vi "大富翁.vi"() -> ()   [LabVIEW 2014] (continued)
                      frame 1, Default {
                        n4206 = local read "玩家一財產"() -> (w3544:dbl)
                      }
                      frame 2 {
                        n4207 = local read "玩家二財產"() -> (w3545:dbl)
                      }
                      frame 3 {
                        n4208 = local read "玩家三財產"() -> (w3546:dbl)
                      }
                      frame 4 {
                        n4209 = local read "玩家四財產"() -> (w3547:dbl)
                      }
                    }
                    n4210 = call "各種價格.vi"("Numeric"=w3516) -> ("買空地"=w3514:dbl)  [unwired: 4 in, 5 out]
                    n4211 = Greater Or Equal?(x=w3515, y=w3514) -> (x >= y?=w3513:bool)
                    n4212 = case shown="True" w3513 {
                      tunnel: w3516 -> [_ w3518]
                      frame False {
                        # "錢不夠"
                        n4213 = call "錢不夠.vi"() -> ()  [unwired: 4 in]
                      }
                      frame True {
                        # "錢夠"
                        n4214 = local read "換誰?"() -> (w3519:dbl)
                        n4215 = case shown="3" w3519 {
                          selector: w3519 -> [w3523 w3529 w3535 w3541]
                          tunnel: w3518 -> [w3522 w3528 w3534 w3540]
                          frame 1, Default {
                            # "誰買了地"
                            n4216 = call "各種價格.vi"("Numeric"=w3522) -> ("買空地"=w3521:dbl)  [unwired: 4 in, 5 out]
                            n4217 = local read "玩家一財產"() -> (w3525:dbl)
                            n4218 = Subtract(x=w3525, y=w3521) -> (x-y=w3524:dbl)
                            n4219 = local write "玩家一財產"(w3524) -> ()
                            n4220 = call "數字轉顏色.vi"("數字"=w3523) -> ("顏色數字"=w3520:dbl)  [unwired: 2 in]
                            n4221 = local write "34新竹縣"(w3520) -> ()
                            n4222 = local write "新竹縣所有"(w3520) -> ()
                          }
                          frame 2 {
                            # "誰買了地"
                            n4223 = call "各種價格.vi"("Numeric"=w3528) -> ("買空地"=w3527:dbl)  [unwired: 4 in, 5 out]
                            n4224 = local read "玩家二財產"() -> (w3531:dbl)
                            n4225 = Subtract(x=w3531, y=w3527) -> (x-y=w3530:dbl)
                            n4226 = local write "玩家二財產"(w3530) -> ()
                            n4227 = call "數字轉顏色.vi"("數字"=w3529) -> ("顏色數字"=w3526:dbl)  [unwired: 2 in]
                            n4228 = local write "34新竹縣"(w3526) -> ()
                            n4229 = local write "新竹縣所有"(w3526) -> ()
                          }
                          frame 3 {
                            # "誰買了地"
                            n4230 = local read "玩家三財產"() -> (w3536:dbl)
                            n4231 = call "各種價格.vi"("Numeric"=w3534) -> ("買空地"=w3533:dbl)  [unwired: 4 in, 5 out]
                            n4232 = Subtract(x=w3536, y=w3533) -> (x-y=w3537:dbl)
                            n4233 = call "數字轉顏色.vi"("數字"=w3535) -> ("顏色數字"=w3532:dbl)  [unwired: 2 in]
                            n4234 = local write "玩家三財產"(w3537) -> ()
                            n4235 = local write "34新竹縣"(w3532) -> ()
                            n4236 = local write "新竹縣所有"(w3532) -> ()
                          }
                          frame 4 {
                            # "誰買了地"
                            n4237 = call "各種價格.vi"("Numeric"=w3540) -> ("買空地"=w3539:dbl)  [unwired: 4 in, 5 out]
                            n4238 = local read "玩家四財產"() -> (w3543:dbl)
                            n4239 = Subtract(x=w3543, y=w3539) -> (x-y=w3542:dbl)
                            n4240 = local write "玩家四財產"(w3542) -> ()
                            n4241 = call "數字轉顏色.vi"("數字"=w3541) -> ("顏色數字"=w3538:dbl)  [unwired: 2 in]
                            n4242 = local write "34新竹縣"(w3538) -> ()
                            n4243 = local write "新竹縣所有"(w3538) -> ()
                          }
                        }
                      }
                    }
                  }
                }
              }
            }
          }
          frame 36 {
            n4244 = local read "新竹市所有"() -> (w3548:u32)
            n4245 = Equal?(x=w3548, y=u32 16777215) -> (x = y?=w3551:bool)
            n4246 = case shown="False" w3551 {
              tunnel: w3550 -> [w3574 w3612]
              tunnel: [w3564 FALSE] -> w3549
              frame False {
                # "有主地"
                n4247 = local read "換誰?"() -> (w3567:dbl)
                n4248 = local read "新竹市所有"() -> (w3555:u32)
                n4249 = call "數字轉顏色.vi"("數字"=w3567) -> ("顏色數字"=w3578:dbl)  [unwired: 2 in]
                n4250 = case shown="4" w3567 {
                  tunnel: [w3607 w3608 w3609 w3610] -> w3573
                  frame 1, Default {
                    n4251 = local read "玩家一財產"() -> (w3607:dbl)
                  }
                  frame 2 {
                    n4252 = local read "玩家二財產"() -> (w3608:dbl)
                  }
                  frame 3 {
                    n4253 = local read "玩家三財產"() -> (w3609:dbl)
                  }
                  frame 4 {
                    n4254 = local read "玩家四財產"() -> (w3610:dbl)
                  }
                }
                n4255 = Equal?(x=w3555, y=w3578) -> (x = y?=w3577:bool)
                n4256 = local read "36旅4"() -> (w3556:bool)
                n4257 = local read "36旅3"() -> (w3557:bool)
                n4258 = local read "36旅2"() -> (w3558:bool)
                n4259 = local read "36旅1"() -> (w3559:bool)
                n4260 = local read "36房4"() -> (w3560:bool)
                n4261 = local read "36房3"() -> (w3561:bool)
                n4262 = local read "36房2"() -> (w3562:bool)
                n4263 = local read "36房1"() -> (w3563:bool)
                n4264 = local read "新竹市所有"() -> (w3554:u32)
                n4265 = call "房子數量.vi"("房子 1"=w3563, "房子 2"=w3562, "房子 3"=w3561, "房子 4"=w3560, "旅館 1"=w3559, "旅館 2"=w3558, "旅館 3"=w3557, "旅館 4"=w3556) -> ("房子數"=w3576:dbl, "旅館數"=w3575:dbl)  [unwired: 18 in]
                n4266 = call "顏色轉數字.vi"("顏色數字"=w3554) -> ("數字"=w3565:dbl)  [unwired: 2 in]
                n4267 = case shown="1, Default" w3565 {
                  tunnel: [w3583 w3584 w3585 w3586] -> w3569
                  frame 1, Default {
                    n4268 = local read "玩家一財產"() -> (w3583:dbl)
                  }
                  frame 2 {
                    n4269 = local read "玩家二財產"() -> (w3584:dbl)
                  }
                  frame 3 {
                    n4270 = local read "玩家三財產"() -> (w3585:dbl)
                  }
                  frame 4 {
                    n4271 = local read "玩家四財產"() -> (w3586:dbl)
                  }
                }
                n4272 = call "走到地.vi"("房子數量"=w3576, "自己的地?"=w3577, "旅館數量"=w3575, "編號"=w3574, "走到人財產"=w3573) -> ("走到人-?"=w3572:dbl, "蓋第幾棟"=w3570:dbl, "地主+?"=w3568:dbl, "破產?"=w3564:bool)
                n4273 = Subtract(x=w3573, y=w3572) -> (x-y=w3571:dbl)
                n4274 = Add(x=w3568, y=w3569) -> (x+y=w3566:dbl)
                n4275 = case shown="1, Default" w3565 {
                  tunnel: w3566 -> [w3579 w3580 w3581 w3582]
                  frame 1, Default {
                    n4276 = local write "玩家一財產"(w3579) -> ()
                  }
                  frame 2 {
                    n4277 = local write "玩家二財產"(w3580) -> ()
                  }
                  frame 3 {
                    n4278 = local write "玩家三財產"(w3581) -> ()
                  }
                  frame 4 {
                    n4279 = local write "玩家四財產"(w3582) -> ()
                  }
                }
                n4280 = case shown="1" w3570 {
                  frame 0, Default {
                  }
                  frame 1 {
                    n4281 = flat-sequence {
                      frame #0 {
                        n4282 = local write "36房1"(TRUE ("1房1")) -> ()
                      }
                      frame #1 {
                        n4283 = property on="36房1" class="Bool (strict)"("Visible"=TRUE) -> ()  [unwired: 2 in, 2 out]
                      }
                    }
                  }
                  frame 2 {
                    n4284 = flat-sequence {
                      frame #0 {
                        n4285 = local write "36房2"(TRUE ("1房2")) -> ()
                      }
                      frame #1 {
                        n4286 = property on="36房2" class="Bool (strict)"("Visible"=TRUE ("1房2")) -> ()  [unwired: 2 in, 2 out]
                      }
                    }
                  }
                  frame 3 {
                    n4287 = flat-sequence {
                      frame #0 {
                        n4288 = local write "36房3"(TRUE) -> ()
                      }
                      frame #1 {
                        n4289 = property on="36房3" class="Bool (strict)"("Visible"=TRUE) -> ()  [unwired: 2 in, 2 out]
                      }
                    }
                  }
                  frame 4 {
                    n4290 = flat-sequence {
                      frame #0 {
                        n4291 = local write "36房4"(TRUE) -> ()
                      }
                      frame #1 {
                        n4292 = property on="36房4" class="Bool (strict)"("Visible"=TRUE) -> ()  [unwired: 2 in, 2 out]
                      }
                    }
                  }
                  frame 5 {
                    n4293 = flat-sequence {
                      frame #0 {
                        n4294 = local write "36旅1"(TRUE) -> ()
                      }
                      frame #1 {
                        n4295 = property on="36旅1" class="Bool (strict)"("Visible"=TRUE) -> ()  [unwired: 2 in, 2 out]
                      }
                    }
                  }
                  frame 6 {
                    n4296 = flat-sequence {
                      frame #0 {
                        n4297 = local write "36旅2"(TRUE) -> ()
                      }
                      frame #1 {
                        n4298 = property on="36旅2" class="Bool (strict)"("Visible"=TRUE) -> ()  [unwired: 2 in, 2 out]
                      }
                    }
                  }
                  frame 7 {
                    n4299 = flat-sequence {
                      frame #0 {
                        n4300 = local write "36旅3"(TRUE) -> ()
                      }
                      frame #1 {
                        n4301 = property on="36旅3" class="Bool (strict)"("Visible"=TRUE) -> ()  [unwired: 2 in, 2 out]
                      }
                    }
                  }
                  frame 8 {
                    n4302 = flat-sequence {
                      frame #0 {
                        n4303 = local write "36旅4"(TRUE) -> ()
                      }
                      frame #1 {
                        n4304 = property on="36旅4" class="Bool (strict)"("Visible"=TRUE) -> ()  [unwired: 2 in, 2 out]
                      }
                    }
                  }
                }
                n4305 = case shown="1, Default" w3567 {
                  tunnel: w3571 -> [w3603 w3604 w3605 w3606]
                  frame 1, Default {
                    n4306 = local write "玩家一財產"(w3603) -> ()
                  }
                  frame 2 {
                    n4307 = local write "玩家二財產"(w3604) -> ()
                  }
                  frame 3 {
                    n4308 = local write "玩家三財產"(w3605) -> ()
                  }
                  frame 4 {
                    n4309 = local write "玩家四財產"(w3606) -> ()
                  }
                }
              }
              frame True {
                # "無主地"
                n4310 = call "購買土地.vi"() -> ("確定 2"=w3613:bool)  [unwired: 3 in]
                n4311 = case shown="True" w3613 {
                  tunnel: w3612 -> [_ w3617]
                  frame False {
                    # "不買"
                  }
                  frame True {
                    # "要買"
                    n4312 = local read "換誰?"() -> (w3618:dbl)
                    n4313 = case shown="4" w3618 {
                      tunnel: [w3645 w3646 w3647 w3648] -> w3616
                      frame 1, Default {
                        n4314 = local read "玩家一財產"() -> (w3645:dbl)
                      }
                      frame 2 {
                        n4315 = local read "玩家二財產"() -> (w3646:dbl)
                      }
                      frame 3 {
                        n4316 = local read "玩家三財產"() -> (w3647:dbl)
                      }
                      frame 4 {
                        n4317 = local read "玩家四財產"() -> (w3648:dbl)
                      }
                    }
                    n4318 = call "各種價格.vi"("Numeric"=w3617) -> ("買空地"=w3615:dbl)  [unwired: 4 in, 5 out]
                    n4319 = Greater Or Equal?(x=w3616, y=w3615) -> (x >= y?=w3614:bool)
                    n4320 = case shown="True" w3614 {
                      tunnel: w3617 -> [_ w3619]
                      frame False {
                        # "錢不夠"
                        n4321 = call "錢不夠.vi"() -> ()  [unwired: 4 in]
                      }
                      frame True {
                        # "錢夠"
                        n4322 = local read "換誰?"() -> (w3620:dbl)
                        n4323 = case shown="4" w3620 {
                          selector: w3620 -> [w3624 w3630 w3636 w3642]
                          tunnel: w3619 -> [w3623 w3629 w3635 w3641]
                          frame 1, Default {
                            # "誰買了地"
                            n4324 = call "各種價格.vi"("Numeric"=w3623) -> ("買空地"=w3622:dbl)  [unwired: 4 in, 5 out]
                            n4325 = local read "玩家一財產"() -> (w3626:dbl)
                            n4326 = Subtract(x=w3626, y=w3622) -> (x-y=w3625:dbl)
                            n4327 = local write "玩家一財產"(w3625) -> ()
                            n4328 = call "數字轉顏色.vi"("數字"=w3624) -> ("顏色數字"=w3621:dbl)  [unwired: 2 in]
                            n4329 = local write "36新竹市"(w3621) -> ()
                            n4330 = local write "新竹市所有"(w3621) -> ()
                          }
                          frame 2 {
                            # "誰買了地"
                            n4331 = call "各種價格.vi"("Numeric"=w3629) -> ("買空地"=w3628:dbl)  [unwired: 4 in, 5 out]
                            n4332 = local read "玩家二財產"() -> (w3632:dbl)
                            n4333 = Subtract(x=w3632, y=w3628) -> (x-y=w3631:dbl)
                            n4334 = local write "玩家二財產"(w3631) -> ()
                            n4335 = call "數字轉顏色.vi"("數字"=w3630) -> ("顏色數字"=w3627:dbl)  [unwired: 2 in]
                            n4336 = local write "36新竹市"(w3627) -> ()
                            n4337 = local write "新竹市所有"(w3627) -> ()
                          }
                          frame 3 {
                            # "誰買了地"
                            n4338 = local read "玩家三財產"() -> (w3637:dbl)
                            n4339 = call "各種價格.vi"("Numeric"=w3635) -> ("買空地"=w3634:dbl)  [unwired: 4 in, 5 out]
                            n4340 = Subtract(x=w3637, y=w3634) -> (x-y=w3638:dbl)
                            n4341 = call "數字轉顏色.vi"("數字"=w3636) -> ("顏色數字"=w3633:dbl)  [unwired: 2 in]
                            n4342 = local write "玩家三財產"(w3638) -> ()
                            n4343 = local write "36新竹市"(w3633) -> ()
                            n4344 = local write "新竹市所有"(w3633) -> ()
                          }
                          frame 4 {
                            # "誰買了地"
                            n4345 = call "各種價格.vi"("Numeric"=w3641) -> ("買空地"=w3640:dbl)  [unwired: 4 in, 5 out]
                            n4346 = local read "玩家四財產"() -> (w3644:dbl)
                            n4347 = Subtract(x=w3644, y=w3640) -> (x-y=w3643:dbl)
                            n4348 = local write "玩家四財產"(w3643) -> ()
                            n4349 = call "數字轉顏色.vi"("數字"=w3642) -> ("顏色數字"=w3639:dbl)  [unwired: 2 in]
                            n4350 = local write "36新竹市"(w3639) -> ()
                            n4351 = local write "新竹市所有"(w3639) -> ()
                          }
                        }
                      }
                    }
                  }
                }
              }
            }
          }
          frame 37 {
            n4352 = local read "中壢市所有"() -> (w3649:u32)
            n4353 = Equal?(x=w3649, y=u32 16777215) -> (x = y?=w3652:bool)
            n4354 = case shown="True" w3652 {
              tunnel: w3651 -> [w3675 w3713]
              tunnel: [w3665 FALSE] -> w3650
              frame False {
                # "有主地"
                n4355 = local read "換誰?"() -> (w3668:dbl)
                n4356 = local read "中壢市所有"() -> (w3656:u32)
                n4357 = call "數字轉顏色.vi"("數字"=w3668) -> ("顏色數字"=w3679:dbl)  [unwired: 2 in]
                n4358 = case shown="4" w3668 {
                  tunnel: [w3708 w3709 w3710 w3711] -> w3674
                  frame 1, Default {
                    n4359 = local read "玩家一財產"() -> (w3708:dbl)
                  }
                  frame 2 {
                    n4360 = local read "玩家二財產"() -> (w3709:dbl)
                  }
                  frame 3 {
                    n4361 = local read "玩家三財產"() -> (w3710:dbl)
                  }
                  frame 4 {
                    n4362 = local read "玩家四財產"() -> (w3711:dbl)
                  }
                }
                n4363 = Equal?(x=w3656, y=w3679) -> (x = y?=w3678:bool)
                n4364 = local read "37旅4"() -> (w3657:bool)
                n4365 = local read "37旅3"() -> (w3658:bool)
                n4366 = local read "37旅2"() -> (w3659:bool)
                n4367 = local read "37旅1"() -> (w3660:bool)
                n4368 = local read "37房4"() -> (w3661:bool)
                n4369 = local read "37房3"() -> (w3662:bool)
                n4370 = local read "37房2"() -> (w3663:bool)
                n4371 = local read "37房1"() -> (w3664:bool)
                n4372 = local read "中壢市所有"() -> (w3655:u32)
                n4373 = call "房子數量.vi"("房子 1"=w3664, "房子 2"=w3663, "房子 3"=w3662, "房子 4"=w3661, "旅館 1"=w3660, "旅館 2"=w3659, "旅館 3"=w3658, "旅館 4"=w3657) -> ("房子數"=w3677:dbl, "旅館數"=w3676:dbl)  [unwired: 18 in]
                n4374 = call "顏色轉數字.vi"("顏色數字"=w3655) -> ("數字"=w3666:dbl)  [unwired: 2 in]
                n4375 = case shown="1, Default" w3666 {
                  tunnel: [w3684 w3685 w3686 w3687] -> w3670
                  frame 1, Default {
                    n4376 = local read "玩家一財產"() -> (w3684:dbl)
                  }
                  frame 2 {
                    n4377 = local read "玩家二財產"() -> (w3685:dbl)
                  }
                  frame 3 {
                    n4378 = local read "玩家三財產"() -> (w3686:dbl)
                  }
                  frame 4 {
                    n4379 = local read "玩家四財產"() -> (w3687:dbl)
                  }
                }
                n4380 = call "走到地.vi"("房子數量"=w3677, "自己的地?"=w3678, "旅館數量"=w3676, "編號"=w3675, "走到人財產"=w3674) -> ("走到人-?"=w3673:dbl, "蓋第幾棟"=w3671:dbl, "地主+?"=w3669:dbl, "破產?"=w3665:bool)
                n4381 = Subtract(x=w3674, y=w3673) -> (x-y=w3672:dbl)
                n4382 = Add(x=w3669, y=w3670) -> (x+y=w3667:dbl)
                n4383 = case shown="1, Default" w3666 {
                  tunnel: w3667 -> [w3680 w3681 w3682 w3683]
                  frame 1, Default {
                    n4384 = local write "玩家一財產"(w3680) -> ()
                  }
                  frame 2 {
                    n4385 = local write "玩家二財產"(w3681) -> ()
                  }
                  frame 3 {
                    n4386 = local write "玩家三財產"(w3682) -> ()
                  }
                  frame 4 {
                    n4387 = local write "玩家四財產"(w3683) -> ()
                  }
                }
                n4388 = case shown="8" w3671 {
                  frame 0, Default {
                  }
                  frame 1 {
                    n4389 = flat-sequence {
                      frame #0 {
                        n4390 = local write "37房1"(TRUE ("1房1")) -> ()
                      }
                      frame #1 {
                        n4391 = property on="37房1" class="Bool (strict)"("Visible"=TRUE) -> ()  [unwired: 2 in, 2 out]
                      }
                    }
                  }
                  frame 2 {
                    n4392 = flat-sequence {
                      frame #0 {
                        n4393 = local write "37房2"(TRUE ("1房2")) -> ()
                      }
                      frame #1 {
                        n4394 = property on="37房2" class="Bool (strict)"("Visible"=TRUE ("1房2")) -> ()  [unwired: 2 in, 2 out]
                      }
                    }
                  }
                  frame 3 {
                    n4395 = flat-sequence {
                      frame #0 {
                        n4396 = local write "37房3"(TRUE) -> ()
                      }
                      frame #1 {
                        n4397 = property on="37房3" class="Bool (strict)"("Visible"=TRUE) -> ()  [unwired: 2 in, 2 out]
                      }
                    }
                  }
                  frame 4 {
                    n4398 = flat-sequence {
                      frame #0 {
                        n4399 = local write "37房4"(TRUE) -> ()
                      }
                      frame #1 {
                        n4400 = property on="37房4" class="Bool (strict)"("Visible"=TRUE) -> ()  [unwired: 2 in, 2 out]
                      }
                    }
                  }
                  frame 5 {
                    n4401 = flat-sequence {
                      frame #0 {
                        n4402 = local write "37旅1"(TRUE) -> ()
                      }
                      frame #1 {
                        n4403 = property on="37旅1" class="Bool (strict)"("Visible"=TRUE) -> ()  [unwired: 2 in, 2 out]
                      }
                    }
                  }
                  frame 6 {
                    n4404 = flat-sequence {
                      frame #0 {
                        n4405 = local write "37旅2"(TRUE) -> ()
                      }
                      frame #1 {
                        n4406 = property on="37旅2" class="Bool (strict)"("Visible"=TRUE) -> ()  [unwired: 2 in, 2 out]
                      }
                    }
                  }
                  frame 7 {
                    n4407 = flat-sequence {
                      frame #0 {
                        n4408 = local write "37旅3"(TRUE) -> ()
                      }
                      frame #1 {
                        n4409 = property on="37旅3" class="Bool (strict)"("Visible"=TRUE) -> ()  [unwired: 2 in, 2 out]
                      }
                    }
                  }
                  frame 8 {
                    n4410 = flat-sequence {
                      frame #0 {
                        n4411 = local write "37旅4"(TRUE) -> ()
                      }
                      frame #1 {
                        n4412 = property on="37旅4" class="Bool (strict)"("Visible"=TRUE) -> ()  [unwired: 2 in, 2 out]
                      }
                    }
                  }
                }
                n4413 = case shown="1, Default" w3668 {
                  tunnel: w3672 -> [w3704 w3705 w3706 w3707]
                  frame 1, Default {
                    n4414 = local write "玩家一財產"(w3704) -> ()
                  }
                  frame 2 {
                    n4415 = local write "玩家二財產"(w3705) -> ()
                  }
                  frame 3 {
                    n4416 = local write "玩家三財產"(w3706) -> ()
                  }
                  frame 4 {
                    n4417 = local write "玩家四財產"(w3707) -> ()
                  }
                }
              }
              frame True {
                # "無主地"
                n4418 = call "購買土地.vi"() -> ("確定 2"=w3714:bool)  [unwired: 3 in]
                n4419 = case shown="True" w3714 {
                  tunnel: w3713 -> [_ w3718]
                  frame False {
                    # "不買"
                  }
                  frame True {
                    # "要買"
                    n4420 = local read "換誰?"() -> (w3719:dbl)
                    n4421 = case shown="4" w3719 {
                      tunnel: [w3746 w3747 w3748 w3749] -> w3717
                      frame 1, Default {
                        n4422 = local read "玩家一財產"() -> (w3746:dbl)
                      }
                      frame 2 {
                        n4423 = local read "玩家二財產"() -> (w3747:dbl)
                      }
                      frame 3 {
                        n4424 = local read "玩家三財產"() -> (w3748:dbl)
                      }
                      frame 4 {
                        n4425 = local read "玩家四財產"() -> (w3749:dbl)
                      }
                    }
                    n4426 = call "各種價格.vi"("Numeric"=w3718) -> ("買空地"=w3716:dbl)  [unwired: 4 in, 5 out]
                    n4427 = Greater Or Equal?(x=w3717, y=w3716) -> (x >= y?=w3715:bool)
                    n4428 = case shown="True" w3715 {
                      tunnel: w3718 -> [_ w3720]
                      frame False {
                        # "錢不夠"
                        n4429 = call "錢不夠.vi"() -> ()  [unwired: 4 in]
                      }
                      frame True {
                        # "錢夠"
                        n4430 = local read "換誰?"() -> (w3721:dbl)
                        n4431 = case shown="3" w3721 {
                          selector: w3721 -> [w3725 w3731 w3737 w3743]
                          tunnel: w3720 -> [w3724 w3730 w3736 w3742]
                          frame 1, Default {
                            # "誰買了地"
                            n4432 = call "各種價格.vi"("Numeric"=w3724) -> ("買空地"=w3723:dbl)  [unwired: 4 in, 5 out]
                            n4433 = local read "玩家一財產"() -> (w3727:dbl)
                            n4434 = Subtract(x=w3727, y=w3723) -> (x-y=w3726:dbl)
                            n4435 = local write "玩家一財產"(w3726) -> ()
                            n4436 = call "數字轉顏色.vi"("數字"=w3725) -> ("顏色數字"=w3722:dbl)  [unwired: 2 in]
                            n4437 = local write "37中壢市"(w3722) -> ()
                            n4438 = local write "中壢市所有"(w3722) -> ()
                          }
                          frame 2 {
                            # "誰買了地"
                            n4439 = call "各種價格.vi"("Numeric"=w3730) -> ("買空地"=w3729:dbl)  [unwired: 4 in, 5 out]
                            n4440 = local read "玩家二財產"() -> (w3733:dbl)
                            n4441 = Subtract(x=w3733, y=w3729) -> (x-y=w3732:dbl)
                            n4442 = local write "玩家二財產"(w3732) -> ()
                            n4443 = call "數字轉顏色.vi"("數字"=w3731) -> ("顏色數字"=w3728:dbl)  [unwired: 2 in]
                            n4444 = local write "37中壢市"(w3728) -> ()
                            n4445 = local write "中壢市所有"(w3728) -> ()
                          }
                          frame 3 {
                            # "誰買了地"
                            n4446 = local read "玩家三財產"() -> (w3738:dbl)
                            n4447 = call "各種價格.vi"("Numeric"=w3736) -> ("買空地"=w3735:dbl)  [unwired: 4 in, 5 out]
                            n4448 = Subtract(x=w3738, y=w3735) -> (x-y=w3739:dbl)
                            n4449 = call "數字轉顏色.vi"("數字"=w3737) -> ("顏色數字"=w3734:dbl)  [unwired: 2 in]
                            n4450 = local write "玩家三財產"(w3739) -> ()
                            n4451 = local write "37中壢市"(w3734) -> ()
                            n4452 = local write "中壢市所有"(w3734) -> ()
                          }
                          frame 4 {
                            # "誰買了地"
                            n4453 = call "各種價格.vi"("Numeric"=w3742) -> ("買空地"=w3741:dbl)  [unwired: 4 in, 5 out]
                            n4454 = local read "玩家四財產"() -> (w3745:dbl)
                            n4455 = Subtract(x=w3745, y=w3741) -> (x-y=w3744:dbl)
                            n4456 = local write "玩家四財產"(w3744) -> ()
                            n4457 = call "數字轉顏色.vi"("數字"=w3743) -> ("顏色數字"=w3740:dbl)  [unwired: 2 in]
                            n4458 = local write "37中壢市"(w3740) -> ()
                            n4459 = local write "中壢市所有"(w3740) -> ()
                          }
                        }
                      }
                    }
                  }
                }
              }
            }
          }
          frame 38 {
            n4460 = stacked-sequence {
              tunnel: [_ _ w3824] -> w3751
              frame #0 {
                w3752 = T1."Disabled" ("Disabled")
                n4461 = property on="擲骰子 4" class="Bool (strict)"("DisabledEnum"=w3752) -> ()  [unwired: 2 in, 2 out]
                n4462 = property on="擲骰子 2" class="Bool (strict)"("DisabledEnum"=w3752) -> ()  [unwired: 2 in, 2 out]
                n4463 = property on="擲骰子 3" class="Bool (strict)"("DisabledEnum"=w3752) -> ()  [unwired: 2 in, 2 out]
                n4464 = property on="擲骰子 1" class="Bool (strict)"("DisabledEnum"=w3752) -> ()  [unwired: 2 in, 2 out]
                n4465 = local write "擲骰子 1"(FALSE ("擲骰子 1")) -> ()
                n4466 = for {
                  N: 70 -> [_]
                  n4467 = call "dice.vi"() -> ("y"=w3755:dbl)  [unwired: 11 in]
                  n4468 = local write "骰子"(w3755) -> ()
                  n4469 = Wait (ms)(milliseconds to wait=u32 10) -> ()  [unwired: 1 out]
                }
              }
              frame #1 {
                n4470 = local read "骰子"() -> (w3757:dbl)
                n4471 = for {
                  N: w3757 -> [_]
                  i -> [w3758]
                  n4472 = local read "位置 1"() -> (w3759:dbl)
                  n4473 = case shown="33..36" w3759 {
                    tunnel: w3758 -> [w3761 _ _ _ _ _ _ _ _ _ _ _]
                    frame 0 {
                      n4474 = Greater Than 0?(x=w3761) -> (x > 0?=w3760:bool)
                      n4475 = case shown="False" w3760 {
                        frame False {
                          n4476 = property on="P1 棋子" class="Bool (strict)"("Left"=300 ("Position:Left")) -> ()  [unwired: 2 in, 2 out]
                          n4477 = local read "位置 1"() -> (w3765:dbl)
                          n4478 = Wait (ms)(milliseconds to wait=u32 700) -> ()  [unwired: 1 out]
                          n4479 = Increment(x=w3765) -> (x+1=w3764:dbl)
                          n4480 = local write "位置 1"(w3764) -> ()
                        }
                        frame True {
                          n4481 = property on="P1 棋子" class="Bool (strict)"("Left"=300 ("Position:Left")) -> ()  [unwired: 2 in, 2 out]
                          n4482 = Wait (ms)(milliseconds to wait=u32 700) -> ()  [unwired: 1 out]
                          n4483 = local read "玩家一財產"() -> (w3770:dbl)
                          n4484 = local read "位置 1"() -> (w3769:dbl)
                          n4485 = Increment(x=w3769) -> (x+1=w3768:dbl)
                          n4486 = Add(x=w3770, y=2000.0) -> (x+y=w3772:dbl)
                          n4487 = local write "位置 1"(w3768) -> ()
                          n4488 = local write "玩家一財產"(w3772) -> ()
                        }
                      }
                    }
                    frame 1..11, Default {
                      n4489 = property on="P1 棋子" class="Bool (strict)"() -> ("Left"=w3778:i32)  [unwired: 2 in, 2 out]
                      n4490 = Add(x=w3778, y=96) -> (x+y=w3777:i32)
                      n4491 = property on="P1 棋子" class="Bool (strict)"("Left"=w3777) -> ()  [unwired: 2 in, 2 out]
                      n4492 = Wait (ms)(milliseconds to wait=u32 700) -> ()  [unwired: 1 out]
                      n4493 = local read "位置 1"() -> (w3776:dbl)
                      n4494 = Increment(x=w3776) -> (x+1=w3775:dbl)
                      n4495 = local write "位置 1"(w3775) -> ()
                    }
                    frame 12 {
                      n4496 = property on="P1 棋子" class="Bool (strict)"("Left"=1503 ("Position:Left")) -> ()  [unwired: 2 in, 2 out]
                      n4497 = Wait (ms)(milliseconds to wait=u32 700) -> ()  [unwired: 1 out]
                      n4498 = local read "位置 1"() -> (w3782:dbl)
                      n4499 = Increment(x=w3782) -> (x+1=w3781:dbl)
                      n4500 = local write "位置 1"(w3781) -> ()
                    }
                    frame 13 {
                      n4501 = property on="P1 棋子" class="Bool (strict)"("Top"=243 ("Position:Top")) -> ()  [unwired: 2 in, 2 out]
                      n4502 = Wait (ms)(milliseconds to wait=u32 700) -> ()  [unwired: 1 out]
                      n4503 = local read "位置 1"() -> (w3786:dbl)
                      n4504 = Increment(x=w3786) -> (x+1=w3785:dbl)
                      n4505 = local write "位置 1"(w3785) -> ()
                    }
                    frame 14..17 {
                      n4506 = property on="P1 棋子" class="Bool (strict)"() -> ("Top"=w3787:i32)  [unwired: 2 in, 2 out]
                      n4507 = Add(x=w3787, y=96) -> (x+y=w3788:i32)
                      n4508 = property on="P1 棋子" class="Bool (strict)"("Top"=w3788) -> ()  [unwired: 2 in, 2 out]
                      n4509 = Wait (ms)(milliseconds to wait=u32 700) -> ()  [unwired: 1 out]
                      n4510 = local read "位置 1"() -> (w3792:dbl)
                      n4511 = Increment(x=w3792) -> (x+1=w3791:dbl)
                      n4512 = local write "位置 1"(w3791) -> ()
                    }
                    frame 18 {
                      n4513 = property on="P1 棋子" class="Bool (strict)"("Top"=766 ("Position:Top")) -> ()  [unwired: 2 in, 2 out]
                      n4514 = Wait (ms)(milliseconds to wait=u32 700) -> ()  [unwired: 1 out]
                      n4515 = local read "位置 1"() -> (w3796:dbl)
                      n4516 = Increment(x=w3796) -> (x+1=w3795:dbl)
                      n4517 = local write "位置 1"(w3795) -> ()
                    }
                    frame 19 {
                      n4518 = property on="P1 棋子" class="Bool (strict)"("Left"=1356 ("Position:Top")) -> ()  [unwired: 2 in, 2 out]
                      n4519 = Wait (ms)(milliseconds to wait=u32 700) -> ()  [unwired: 1 out]
                      n4520 = local read "位置 1"() -> (w3800:dbl)
                      n4521 = Increment(x=w3800) -> (x+1=w3799:dbl)
                      n4522 = local write "位置 1"(w3799) -> ()
                    }
                    frame 20..30 {
                      n4523 = property on="P1 棋子" class="Bool (strict)"() -> ("Left"=w3803:i32)  [unwired: 2 in, 2 out]
                      n4524 = Subtract(x=w3803, y=96) -> (x-y=w3802:i32)
                      n4525 = property on="P1 棋子" class="Bool (strict)"("Left"=w3802) -> ()  [unwired: 2 in, 2 out]
                      n4526 = Wait (ms)(milliseconds to wait=u32 700) -> ()  [unwired: 1 out]
                      n4527 = local read "位置 1"() -> (w3806:dbl)
                      n4528 = Increment(x=w3806) -> (x+1=w3805:dbl)
                      n4529 = local write "位置 1"(w3805) -> ()
                    }
                    frame 31 {
                      n4530 = property on="P1 棋子" class="Bool (strict)"("Left"=160 ("Position:Top")) -> ()  [unwired: 2 in, 2 out]
                      n4531 = Wait (ms)(milliseconds to wait=u32 700) -> ()  [unwired: 1 out]
                      n4532 = local read "位置 1"() -> (w3810:dbl)
                      n4533 = Increment(x=w3810) -> (x+1=w3809:dbl)
                      n4534 = local write "位置 1"(w3809) -> ()
                    }
                    frame 32 {
                      n4535 = property on="P1 棋子" class="Bool (strict)"("Top"=627 ("Position:Top")) -> ()  [unwired: 2 in, 2 out]
                      n4536 = Wait (ms)(milliseconds to wait=u32 700) -> ()  [unwired: 1 out]
                      n4537 = local read "位置 1"() -> (w3814:dbl)
                      n4538 = Increment(x=w3814) -> (x+1=w3813:dbl)
                      n4539 = local write "位置 1"(w3813) -> ()
                    }
                    frame 33..36 {
                      n4540 = property on="P1 棋子" class="Bool (strict)"() -> ("Top"=w3815:i32)  [unwired: 2 in, 2 out]
                      n4541 = Subtract(x=w3815, y=96) -> (x-y=w3816:i32)
                      n4542 = property on="P1 棋子" class="Bool (strict)"("Top"=w3816) -> ()  [unwired: 2 in, 2 out]
                      n4543 = Wait (ms)(milliseconds to wait=u32 700) -> ()  [unwired: 1 out]
                      n4544 = local read "位置 1"() -> (w3820:dbl)
                      n4545 = Increment(x=w3820) -> (x+1=w3819:dbl)
                      n4546 = local write "位置 1"(w3819) -> ()
                    }
                    frame 37 {
                      n4547 = property on="P1 棋子" class="Bool (strict)"("Top"=112 ("Position:Top")) -> ()  [unwired: 2 in, 2 out]
                      n4548 = Wait (ms)(milliseconds to wait=u32 700) -> ()  [unwired: 1 out]
                      n4549 = local write "位置 1"(0.0 ("位置 1")) -> ()
                    }
                  }
                }
              }
              frame #2 {
                n4550 = local read "位置 1"() -> (w3824:dbl)
              }
            }
          }
          frame 39 {
            n4551 = stacked-sequence {
              tunnel: [_ _ w3899] -> w3826
              frame #0 {
                w3827 = T1."Disabled" ("Disabled")
                n4552 = property on="擲骰子 4" class="Bool (strict)"("DisabledEnum"=w3827) -> ()  [unwired: 2 in, 2 out]
                n4553 = property on="擲骰子 2" class="Bool (strict)"("DisabledEnum"=w3827) -> ()  [unwired: 2 in, 2 out]
                n4554 = property on="擲骰子 3" class="Bool (strict)"("DisabledEnum"=w3827) -> ()  [unwired: 2 in, 2 out]
                n4555 = property on="擲骰子 1" class="Bool (strict)"("DisabledEnum"=w3827) -> ()  [unwired: 2 in, 2 out]
                n4556 = for {
                  N: 70 -> [_]
                  n4557 = call "dice.vi"() -> ("y"=w3830:dbl)  [unwired: 11 in]
                  n4558 = local write "骰子"(w3830) -> ()
                  n4559 = Wait (ms)(milliseconds to wait=u32 10) -> ()  [unwired: 1 out]
                }
                n4560 = local write "擲骰子 2"(FALSE ("擲骰子 1")) -> ()
              }
              frame #1 {
                n4561 = local read "骰子"() -> (w3832:dbl)
                n4562 = for {
                  N: w3832 -> [_]
                  i -> [w3834]
                  n4563 = local read "位置 2"() -> (w3833:dbl)
                  n4564 = case shown="31" w3833 {
                    tunnel: w3834 -> [w3836 _ _ _ _ _ _ _ _ _ _ _]
                    frame 0 {
                      n4565 = Greater Than 0?(x=w3836) -> (x > 0?=w3835:bool)
                      n4566 = case shown="False" w3835 {
                        frame False {
                          n4567 = property on="P2 棋子" class="Bool (strict)"("Left"=337 ("Position:Left")) -> ()  [unwired: 2 in, 2 out]
                          n4568 = Wait (ms)(milliseconds to wait=u32 700) -> ()  [unwired: 1 out]
                          n4569 = local read "位置 2"() -> (w3837:dbl)
                          n4570 = Increment(x=w3837) -> (x+1=w3838:dbl)
                          n4571 = local write "位置 2"(w3838) -> ()
                        }
                        frame True {
                          n4572 = property on="P2 棋子" class="Bool (strict)"("Left"=337 ("Position:Left")) -> ()  [unwired: 2 in, 2 out]
                          n4573 = Wait (ms)(milliseconds to wait=u32 700) -> ()  [unwired: 1 out]
                          n4574 = local read "玩家二財產"() -> (w3842:dbl)
                          n4575 = local read "位置 2"() -> (w3843:dbl)
                          n4576 = Increment(x=w3843) -> (x+1=w3844:dbl)
                          n4577 = Add(x=w3842, y=2000.0) -> (x+y=w3841:dbl)
                          n4578 = local write "位置 2"(w3844) -> ()
                          n4579 = local write "玩家二財產"(w3841) -> ()
                        }
                      }
                    }
                    frame 1..11, Default {
                      n4580 = property on="P2 棋子" class="Bool (strict)"() -> ("Left"=w3851:i32)  [unwired: 2 in, 2 out]
                      n4581 = Add(x=w3851, y=96) -> (x+y=w3850:i32)
                      n4582 = property on="P2 棋子" class="Bool (strict)"("Left"=w3850) -> ()  [unwired: 2 in, 2 out]
                      n4583 = Wait (ms)(milliseconds to wait=u32 700) -> ()  [unwired: 1 out]
                      n4584 = local read "位置 2"() -> (w3848:dbl)
                      n4585 = Increment(x=w3848) -> (x+1=w3849:dbl)
                      n4586 = local write "位置 2"(w3849) -> ()
                    }
                    frame 12 {
                      n4587 = property on="P2 棋子" class="Bool (strict)"("Left"=1540 ("Position:Left")) -> ()  [unwired: 2 in, 2 out]
                      n4588 = Wait (ms)(milliseconds to wait=u32 700) -> ()  [unwired: 1 out]
                      n4589 = local read "位置 2"() -> (w3855:dbl)
                      n4590 = Increment(x=w3855) -> (x+1=w3854:dbl)
                      n4591 = local write "位置 2"(w3854) -> ()
                    }
                    frame 13 {
                      n4592 = property on="P2 棋子" class="Bool (strict)"("Top"=243 ("Position:Top")) -> ()  [unwired: 2 in, 2 out]
                      n4593 = Wait (ms)(milliseconds to wait=u32 700) -> ()  [unwired: 1 out]
                      n4594 = local read "位置 2"() -> (w3860:dbl)
                      n4595 = Increment(x=w3860) -> (x+1=w3859:dbl)
                      n4596 = local write "位置 2"(w3859) -> ()
                    }
                    frame 14..17 {
                      n4597 = property on="P2 棋子" class="Bool (strict)"() -> ("Top"=w3865:i32)  [unwired: 2 in, 2 out]
                      n4598 = Add(x=w3865, y=96) -> (x+y=w3864:i32)
                      n4599 = property on="P2 棋子" class="Bool (strict)"("Top"=w3864) -> ()  [unwired: 2 in, 2 out]
                      n4600 = Wait (ms)(milliseconds to wait=u32 700) -> ()  [unwired: 1 out]
                      n4601 = local read "位置 2"() -> (w3863:dbl)
                      n4602 = Increment(x=w3863) -> (x+1=w3862:dbl)
                      n4603 = local write "位置 2"(w3862) -> ()
                    }
                    frame 18 {
                      n4604 = property on="P2 棋子" class="Bool (strict)"("Top"=766 ("Position:Top")) -> ()  [unwired: 2 in, 2 out]
                      n4605 = Wait (ms)(milliseconds to wait=u32 700) -> ()  [unwired: 1 out]
                      n4606 = local read "位置 2"() -> (w3868:dbl)
                      n4607 = Increment(x=w3868) -> (x+1=w3869:dbl)
                      n4608 = local write "位置 2"(w3869) -> ()
                    }
                    frame 19 {
                      n4609 = property on="P2 棋子" class="Bool (strict)"("Left"=1393 ("Position:Top")) -> ()  [unwired: 2 in, 2 out]
                      n4610 = Wait (ms)(milliseconds to wait=u32 700) -> ()  [unwired: 1 out]
                      n4611 = local read "位置 2"() -> (w3872:dbl)
                      n4612 = Increment(x=w3872) -> (x+1=w3873:dbl)
                      n4613 = local write "位置 2"(w3873) -> ()
                    }
                    frame 20..30 {
                      n4614 = property on="P2 棋子" class="Bool (strict)"() -> ("Left"=w3878:i32)  [unwired: 2 in, 2 out]
                      n4615 = Subtract(x=w3878, y=96) -> (x-y=w3879:i32)
                      n4616 = property on="P2 棋子" class="Bool (strict)"("Left"=w3879) -> ()  [unwired: 2 in, 2 out]
                      n4617 = Wait (ms)(milliseconds to wait=u32 700) -> ()  [unwired: 1 out]
                      n4618 = local read "位置 2"() -> (w3876:dbl)
                      n4619 = Increment(x=w3876) -> (x+1=w3877:dbl)
                      n4620 = local write "位置 2"(w3877) -> ()
                    }
                    frame 31 {
                      n4621 = property on="P2 棋子" class="Bool (strict)"("Left"=197 ("Position:Top")) -> ()  [unwired: 2 in, 2 out]
                      n4622 = Wait (ms)(milliseconds to wait=u32 700) -> ()  [unwired: 1 out]
                      n4623 = local read "位置 2"() -> (w3883:dbl)
                      n4624 = Increment(x=w3883) -> (x+1=w3882:dbl)
                      n4625 = local write "位置 2"(w3882) -> ()
                    }
                    frame 32 {
                      n4626 = property on="P2 棋子" class="Bool (strict)"("Top"=627 ("Position:Top")) -> ()  [unwired: 2 in, 2 out]
                      n4627 = Wait (ms)(milliseconds to wait=u32 700) -> ()  [unwired: 1 out]
                      n4628 = local read "位置 2"() -> (w3886:dbl)
                      n4629 = Increment(x=w3886) -> (x+1=w3887:dbl)
                      n4630 = local write "位置 2"(w3887) -> ()
                    }
                    frame 33..36 {
                      n4631 = property on="P2 棋子" class="Bool (strict)"() -> ("Top"=w3893:i32)  [unwired: 2 in, 2 out]
                      n4632 = Subtract(x=w3893, y=96) -> (x-y=w3892:i32)
                      n4633 = property on="P2 棋子" class="Bool (strict)"("Top"=w3892) -> ()  [unwired: 2 in, 2 out]
                      n4634 = Wait (ms)(milliseconds to wait=u32 700) -> ()  [unwired: 1 out]
                      n4635 = local read "位置 2"() -> (w3890:dbl)
                      n4636 = Increment(x=w3890) -> (x+1=w3891:dbl)
                      n4637 = local write "位置 2"(w3891) -> ()
                    }
                    frame 37 {
                      n4638 = property on="P2 棋子" class="Bool (strict)"("Top"=112 ("Position:Top")) -> ()  [unwired: 2 in, 2 out]
                      n4639 = Wait (ms)(milliseconds to wait=u32 700) -> ()  [unwired: 1 out]
                      n4640 = local write "位置 2"(0.0 ("位置 2")) -> ()
                    }
                  }
                }
              }
              frame #2 {
                n4641 = local read "位置 2"() -> (w3899:dbl)
              }
            }
          }
          frame 40 {
            n4642 = stacked-sequence {
              tunnel: [_ _ w3974] -> w3901
              frame #0 {
                w3902 = T1."Disabled" ("Disabled")
                n4643 = property on="擲骰子 4" class="Bool (strict)"("DisabledEnum"=w3902) -> ()  [unwired: 2 in, 2 out]
                n4644 = property on="擲骰子 2" class="Bool (strict)"("DisabledEnum"=w3902) -> ()  [unwired: 2 in, 2 out]
                n4645 = property on="擲骰子 3" class="Bool (strict)"("DisabledEnum"=w3902) -> ()  [unwired: 2 in, 2 out]
                n4646 = property on="擲骰子 1" class="Bool (strict)"("DisabledEnum"=w3902) -> ()  [unwired: 2 in, 2 out]
                n4647 = for {
                  N: 70 -> [_]
                  n4648 = call "dice.vi"() -> ("y"=w3905:dbl)  [unwired: 11 in]
                  n4649 = local write "骰子"(w3905) -> ()
                  n4650 = Wait (ms)(milliseconds to wait=u32 10) -> ()  [unwired: 1 out]
                }
                n4651 = local write "擲骰子 3"(FALSE ("擲骰子 3")) -> ()
              }
              frame #1 {
                n4652 = local read "骰子"() -> (w3907:dbl)
                n4653 = for {
                  N: w3907 -> [_]
                  i -> [w3909]
                  n4654 = local read "位置 3"() -> (w3908:dbl)
                  n4655 = case shown="32" w3908 {
                    tunnel: w3909 -> [w3911 _ _ _ _ _ _ _ _ _ _ _]
                    frame 0 {
                      n4656 = Greater Than 0?(x=w3911) -> (x > 0?=w3910:bool)
                      n4657 = case shown="False" w3910 {
                        frame False {
                          n4658 = property on="P3 棋子" class="Bool (strict)"("Left"=300 ("Position:Left")) -> ()  [unwired: 2 in, 2 out]
                          n4659 = local read "位置 3"() -> (w3913:dbl)
                          n4660 = Wait (ms)(milliseconds to wait=u32 700) -> ()  [unwired: 1 out]
                          n4661 = Increment(x=w3913) -> (x+1=w3912:dbl)
                          n4662 = local write "位置 3"(w3912) -> ()
                        }
                        frame True {
                          n4663 = property on="P3 棋子" class="Bool (strict)"("Left"=300 ("Position:Left")) -> ()  [unwired: 2 in, 2 out]
                          n4664 = Wait (ms)(milliseconds to wait=u32 700) -> ()  [unwired: 1 out]
                          n4665 = local read "玩家三財產"() -> (w3916:dbl)
                          n4666 = local read "位置 3"() -> (w3919:dbl)
                          n4667 = Increment(x=w3919) -> (x+1=w3918:dbl)
                          n4668 = Add(x=w3916, y=2000.0) -> (x+y=w3917:dbl)
                          n4669 = local write "玩家三財產"(w3917) -> ()
                          n4670 = local write "位置 3"(w3918) -> ()
                        }
                      }
                    }
                    frame 1..11, Default {
                      n4671 = property on="P3 棋子" class="Bool (strict)"() -> ("Left"=w3925:i32)  [unwired: 2 in, 2 out]
                      n4672 = Add(x=w3925, y=96) -> (x+y=w3926:i32)
                      n4673 = property on="P3 棋子" class="Bool (strict)"("Left"=w3926) -> ()  [unwired: 2 in, 2 out]
                      n4674 = Wait (ms)(milliseconds to wait=u32 700) -> ()  [unwired: 1 out]
                      n4675 = local read "位置 3"() -> (w3924:dbl)
                      n4676 = Increment(x=w3924) -> (x+1=w3923:dbl)
                      n4677 = local write "位置 3"(w3923) -> ()
                    }
                    frame 12 {
                      n4678 = property on="P3 棋子" class="Bool (strict)"("Left"=1503 ("Position:Left")) -> ()  [unwired: 2 in, 2 out]
                      n4679 = Wait (ms)(milliseconds to wait=u32 700) -> ()  [unwired: 1 out]
                      n4680 = local read "位置 3"() -> (w3930:dbl)
                      n4681 = Increment(x=w3930) -> (x+1=w3929:dbl)
                      n4682 = local write "位置 3"(w3929) -> ()
                    }
                    frame 13 {
                      n4683 = property on="P3 棋子" class="Bool (strict)"("Top"=275 ("Position:Top")) -> ()  [unwired: 2 in, 2 out]
                      n4684 = Wait (ms)(milliseconds to wait=u32 700) -> ()  [unwired: 1 out]
                      n4685 = local read "位置 3"() -> (w3934:dbl)
                      n4686 = Increment(x=w3934) -> (x+1=w3933:dbl)
                      n4687 = local write "位置 3"(w3933) -> ()
                    }
                    frame 14..17 {
                      n4688 = property on="P3 棋子" class="Bool (strict)"() -> ("Top"=w3939:i32)  [unwired: 2 in, 2 out]
                      n4689 = Add(x=w3939, y=96) -> (x+y=w3940:i32)
                      n4690 = property on="P3 棋子" class="Bool (strict)"("Top"=w3940) -> ()  [unwired: 2 in, 2 out]
                      n4691 = Wait (ms)(milliseconds to wait=u32 700) -> ()  [unwired: 1 out]
                      n4692 = local read "位置 3"() -> (w3938:dbl)
                      n4693 = Increment(x=w3938) -> (x+1=w3937:dbl)
                      n4694 = local write "位置 3"(w3937) -> ()
                    }
                    frame 18 {
                      n4695 = property on="P3 棋子" class="Bool (strict)"("Top"=798 ("Position:Top")) -> ()  [unwired: 2 in, 2 out]
                      n4696 = Wait (ms)(milliseconds to wait=u32 700) -> ()  [unwired: 1 out]
                      n4697 = local read "位置 3"() -> (w3944:dbl)
                      n4698 = Increment(x=w3944) -> (x+1=w3943:dbl)
                      n4699 = local write "位置 3"(w3943) -> ()
                    }
                    frame 19 {
                      n4700 = property on="P3 棋子" class="Bool (strict)"("Left"=1356 ("Position:Top")) -> ()  [unwired: 2 in, 2 out]
                      n4701 = Wait (ms)(milliseconds to wait=u32 700) -> ()  [unwired: 1 out]
                      n4702 = local read "位置 3"() -> (w3948:dbl)
                      n4703 = Increment(x=w3948) -> (x+1=w3947:dbl)
                      n4704 = local write "位置 3"(w3947) -> ()
                    }
                    frame 20..30 {
                      n4705 = property on="P3 棋子" class="Bool (strict)"() -> ("Left"=w3952:i32)  [unwired: 2 in, 2 out]
                      n4706 = Subtract(x=w3952, y=96) -> (x-y=w3951:i32)
                      n4707 = property on="P3 棋子" class="Bool (strict)"("Left"=w3951) -> ()  [unwired: 2 in, 2 out]
                      n4708 = Wait (ms)(milliseconds to wait=u32 700) -> ()  [unwired: 1 out]
                      n4709 = local read "位置 3"() -> (w3954:dbl)
                      n4710 = Increment(x=w3954) -> (x+1=w3953:dbl)
                      n4711 = local write "位置 3"(w3953) -> ()
                    }
                    frame 31 {
                      n4712 = property on="P3 棋子" class="Bool (strict)"("Left"=160 ("Position:Top")) -> ()  [unwired: 2 in, 2 out]
                      n4713 = Wait (ms)(milliseconds to wait=u32 700) -> ()  [unwired: 1 out]
                      n4714 = local read "位置 3"() -> (w3959:dbl)
                      n4715 = Increment(x=w3959) -> (x+1=w3958:dbl)
                      n4716 = local write "位置 3"(w3958) -> ()
                    }
                    frame 32 {
                      n4717 = property on="P3 棋子" class="Bool (strict)"("Top"=659 ("Position:Top")) -> ()  [unwired: 2 in, 2 out]
                      n4718 = Wait (ms)(milliseconds to wait=u32 700) -> ()  [unwired: 1 out]
